vi "find_template.vi"(5 "Shrink Factor":i32=1, 6 "Field of View":cluster{"fieldOfViewX":sgl, "fieldOfViewY":sgl}, 8 "error in":errorcluster, 10 "find_template parameters":T2, 11 "Image":T3) -> (0 "error out":errorcluster, 2 "Matches":T1(array[cluster]))   [LabVIEW 2024, in "Vision.lvlib"]
uses:
  Vision.lvlib
  <vilib>/vision/Image Controls.llb/IMAQ Image.ctl
  find_template parameters.ctl
  bin/PatternRecognition.dll
panel:
  # "Image must be an 8-bin greyscale image"
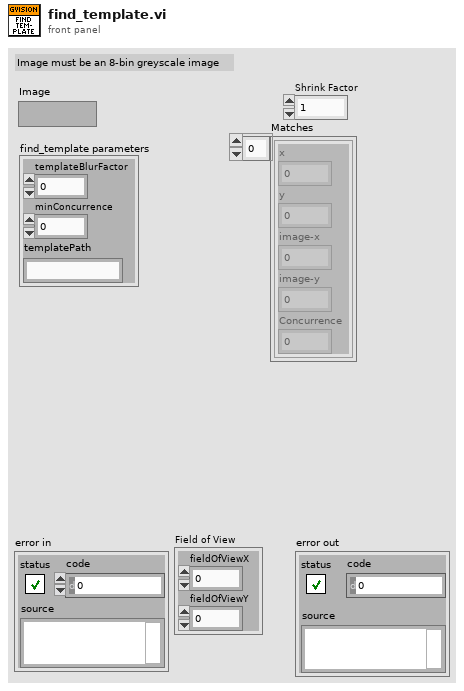
[diagram p1: front panel]
types:
  T1 = cluster{"x":dbl, "y":dbl, "image-x":dbl, "image-y":dbl, "Concurrence":dbl}[]
  T2 = typedef "Vision.lvlib/find_template parameters.ctl" = cluster{"templateBlurFactor":i32, "minConcurrence":sgl, "templatePath":string}
  T3 = typedef "IMAQ Image.ctl" = refnum<image>
  T4 = enum32{"Map Pixel Pointer", "Unmap Pixel Pointer", "Get Pixels Infos"}
  T5 = cluster{"x":dbl, "y":dbl, "image-x":dbl, "image-y":dbl, "Concurrence":dbl}
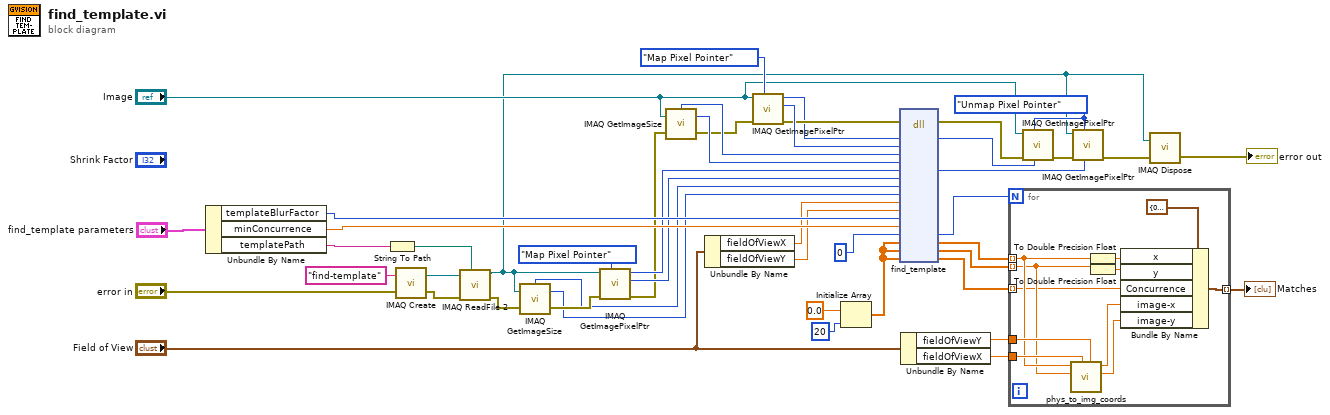
[diagram p0: block diagram]
diagram:
  w7 = T4."Unmap Pixel Pointer" ("Function")
  n1 = Unbundle By Name("find_template parameters") -> ("templateBlurFactor"=w41:i32, "minConcurrence"=w40:sgl, "templatePath"=w21:string)
  n2 = String To Path(string=w21) -> (path=w20:path)
  n3 = call "IMAQ Create"("Image Name"="find-template", "error in (no error)"="error in") -> ("New Image"=w25:T3, "error out"=w24:errorcluster)  [unwired: 3 in]
  n4 = call "IMAQ ReadFile 2"("File Path"=w20, "error in (no error)"=w24, "Image"=w25) -> ("error out"=w13:errorcluster, "Image Out"=w1:T3)  [unwired: 4 in, 3 out]
  n5 = call "IMAQ GetImageSize"("Image"=w1, "error in (no error)"=w13) -> ("Y Resolution"=w14:i32, "X Resolution"=w15:i32, "error out"=w18:errorcluster)  [unwired: 2 in]
  n6 = call "IMAQ GetImagePixelPtr"("Function"=T4."Map Pixel Pointer", "error in (no error)"=w18, "Image"=w1) -> ("error out"=w12:errorcluster, "LineWidth(Pixels)"=w16:i32, "Pixel Pointer out"=w17:u64)  [unwired: 3 in, 3 out]
  n7 = call "IMAQ GetImageSize"("Image"="Image", "error in (no error)"=w12) -> ("Y Resolution"=w33:i32, "X Resolution"=w34:i32, "error out"=w32:errorcluster)  [unwired: 2 in]
  n8 = Unbundle By Name("Field of View") -> ("fieldOfViewX"=w28:sgl, "fieldOfViewY"=w27:sgl)
  n9 = call "IMAQ GetImagePixelPtr"("Function"=T4."Map Pixel Pointer", "error in (no error)"=w32, "Image"="Image") -> ("error out"=w35:errorcluster, "LineWidth(Pixels)"=w43:i32, "Pixel Pointer out"=w6:u64)  [unwired: 3 in, 3 out]
  n10 = Initialize Array(sgl 0.0 ("element"), 20 ("dimension size")) -> (w39:sgl[])
  n11 = dll-call lib="C:/Users/cfang/Desktop/nebraska-silicon-lab/pixel-gantry-control/Gantry/Shared Components/bin/PatternRecognition.dll" fn="find_template"(error in=w35, "imgPtr"=w6, "imgLineWidth"=w43, "imgWidth"=w34, "imgHeight"=w33, "templatePtr"=w17, "templateLineWidth"=w16, "templateWidth"=w15, "templateHeight"=w14, "fieldOfViewX"=w28, "fieldOfViewY"=w27, "templateBlurFactor"=w41, "minConcurrence"=w40, "numMatch"=0 ("numFiducials"), "matchX"=w39, "matchY"=w39, "matchConcurrance"=w39) -> (error out=w10:errorcluster, "imgPtr"=w5:u64, "templatePtr"=w4:u64, "numMatch"=w42:i32, "matchX"=w38:sgl[], "matchY"=w37:sgl[], "matchConcurrance"=w36:sgl[])  [unwired: 13 in, 1 out]
  n12 = Unbundle By Name("Field of View") -> ("fieldOfViewY"=w31:sgl, "fieldOfViewX"=w30:sgl)
  n13 = for {
    N: w42 -> [_]
    tunnel: w38 -> [w52] mode=indexing
    tunnel: w37 -> [w51] mode=indexing
    tunnel: [w58] -> w11 mode=indexing
    tunnel: w36 -> [w48] mode=indexing
    tunnel: w31 -> [w54]
    tunnel: w30 -> [w53]
    n14 = call "phys_to_img_coords.vi"("fov_y"=w54, "fov_x"=w53, "y"=w51, "x"=w52) -> ("image_y"=w49:dbl, "image_x"=w50:dbl)  [unwired: 6 in]
    n15 = To Double Precision Float(number=w52) -> (double precision float=w57:dbl)
    n16 = To Double Precision Float(number=w51) -> (double precision float=w56:dbl)
    n17 = Bundle By Name(cluster=T5 {"x"=0.0, "y"=0.0, "image-x"=0.0, "image-y"=0.0, "Concurrence"=0.0}, "x"=w57, "y"=w56, "Concurrence"=w48, "image-x"=w50, "image-y"=w49) -> (w58:T5)
  }
  "Matches" <- w11
  n18 = call "IMAQ GetImagePixelPtr"("Pixel Pointer in"=w5, "Function"=w7, "error in (no error)"=w10, "Image"="Image") -> ("error out"=w9:errorcluster)  [unwired: 2 in, 5 out]
  n19 = call "IMAQ GetImagePixelPtr"("Pixel Pointer in"=w4, "Function"=w7, "error in (no error)"=w9, "Image"=w1) -> ("error out"=w8:errorcluster)  [unwired: 2 in, 5 out]
  n20 = call "IMAQ Dispose"("Image"=w1, "error in (no error)"=w8) -> ("error out"=→"error out":errorcluster)  [unwired: 4 in]
